vi "Remove Zeros By Interpolation [DBL].vi"(8 "Error In":errorcluster, 11 "Array in":dbl[](array[numeric])) -> (0 "Error Out":errorcluster, 3 "Array out":dbl[](array[numeric]))   [LabVIEW 2019]
doc: "Replaces zero elements by an interpolated value between the nearest non-zero elements.\nRepeats until there is no zero elements left or there is no change from one iteration to the next (in which case an error is returned)."
uses:
  <vilib>/Utility/error.llb/Error Cluster From Error Code.vi
  <vilib>/ErrorRing/Error Ring.xnode
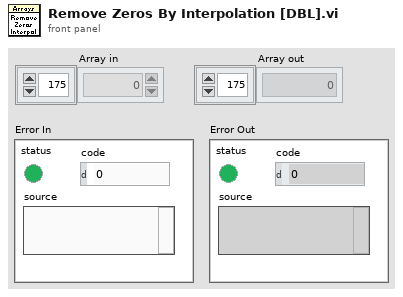
[diagram p1: front panel]
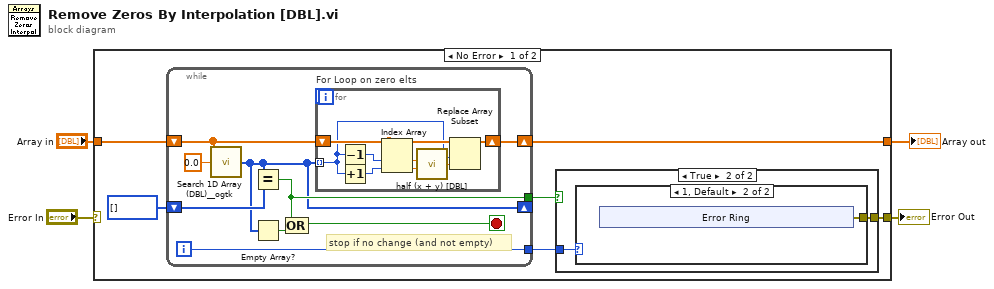
[diagram p0: block diagram]
diagram:
  n1 = case shown="No Error" "Error In" {
    selector: "Error In" -> [_ w36]
    tunnel: "Array in" -> [w9 w35]
    tunnel: [w10 w36] -> w3
    tunnel: [w8 w35] -> w1
    frame No Error {
      n2 = while {
        shift-right: [w24] -> w8
        shift-left: w9 -> [w25]
        shift-right: [w19] -> _
        shift-left: i32[] [] ("Indices of Elements") -> [w23]
        tunnel: [w20] -> w7
        tunnel: [w18] -> w5
        i -> [w18]
        stop <- w22 stop-if-true
        # "stop if no change (and not empty)"
        n3 = call <userlib>:"Search 1D Array (DBL)__ogtk.vi"("Array"=w25, "Element Data"=0.0) -> ("Indices of Elements"=w19:i32[])  [unwired: 7 in]
        n4 = Equal?(x=w19, y=w23) -> (x = y?=w20:bool)
        n5 = Empty Array?(array=w19) -> (empty?=w21:bool)
        n6 = Compound Arithmetic op=OR(w20, w21) -> (w22:bool)
        n7 = for "For Loop on zero elts" {
          tunnel: w19 -> [w28] mode=indexing
          shift-right: [w27] -> w24
          shift-left: w25 -> [w30]
          n8 = Decrement(x=w28) -> (x-1=w34:i32)
          n9 = Increment(x=w28) -> (x+1=w33:i32)
          n10 = Index Array(array=w30, index #1=w34, index #2=w33) -> (element #1=w32:dbl, element #2=w31:dbl)
          n11 = call "half (x + y) [DBL].vi"("y"=w31, "x"=w32) -> ("(x+y)/2"=w29:dbl)  [unwired: 4 in]
          n12 = Replace Array Subset(array=w30, new element=w29, index=w28) -> (w27:dbl[])
        }
      }
      n13 = case shown="True" w7 {
        tunnel: [_ w12] -> w10
        tunnel: w5 -> [_ w11]
        frame False {
        }
        frame True {
          n14 = case shown="1, Default" w11 {
            tunnel: [_ w13] -> w12
            frame 0 {
            }
            frame 1, Default {
              n15 = xnode "Error Ring"() -> ("error out"=w13:errorcluster)
            }
          }
        }
      }
    }
    frame Error {
    }
  }
  "Error Out" <- w3
  "Array out" <- w1
